vi "Send Text Using SMTP API 2013 NIVerified.vi"(2 "phone number 2":string, 3 "Carrier 2":enum16{"T-Mobile", "AT&T", "Verizon", "Sprint"}(ring), 4 "Body":string, 5 "Carrier 1":enum16{"T-Mobile", "AT&T", "Verizon", "Sprint"}(ring), 6 "Subject":string, 7 "phone number 1":string, 9 "Outgoing Mail Server (SMTP)":string="smtp.gmail.com", 10 "Password":string, 11 "Email":string) -> ()   [LabVIEW 2018]
uses:
  <vilib>/smtpClient/Set Message Text.vi
  <vilib>/smtpClient/LabVIEWSMTPClient.lvlib
panel:
  in  "TLS":bool=TRUE
  # "Overview\nThis example will allows you to use an SMTP server to send a SMS message to a cell phone.\nDescription\nWith the SMTP API you can send an email to your phone as a text message.  There are a lot of different servers you\n can use the default in this example is using GMAIL through the smtp.gmail.com server.  Most SMTP servers should \nwork, but the server and cell phone needs to be compatible to send and receive SMS messages.\nSteps to Implement or Execute Code\nOpen Send Text using SMTP API.vi\nFill in the SMTP server in the Outgoing Mail Server (SMTP), gmail is the default server\nFill out your email & Password\nSelect your Carrier and Type your Phone Number\nType the text you would like to send in the Body Control"
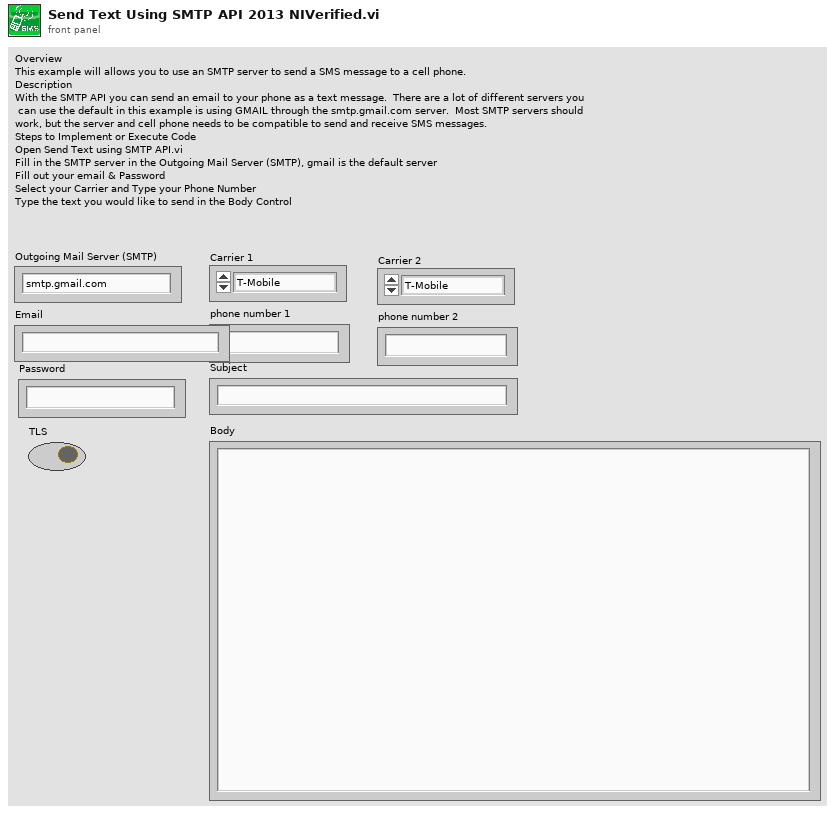
[diagram p1: front panel]
types:
  T1 = typedef "LabVIEWSMTPClient.lvlib/SmtpClientHandle.ctl" = refnum<k1>
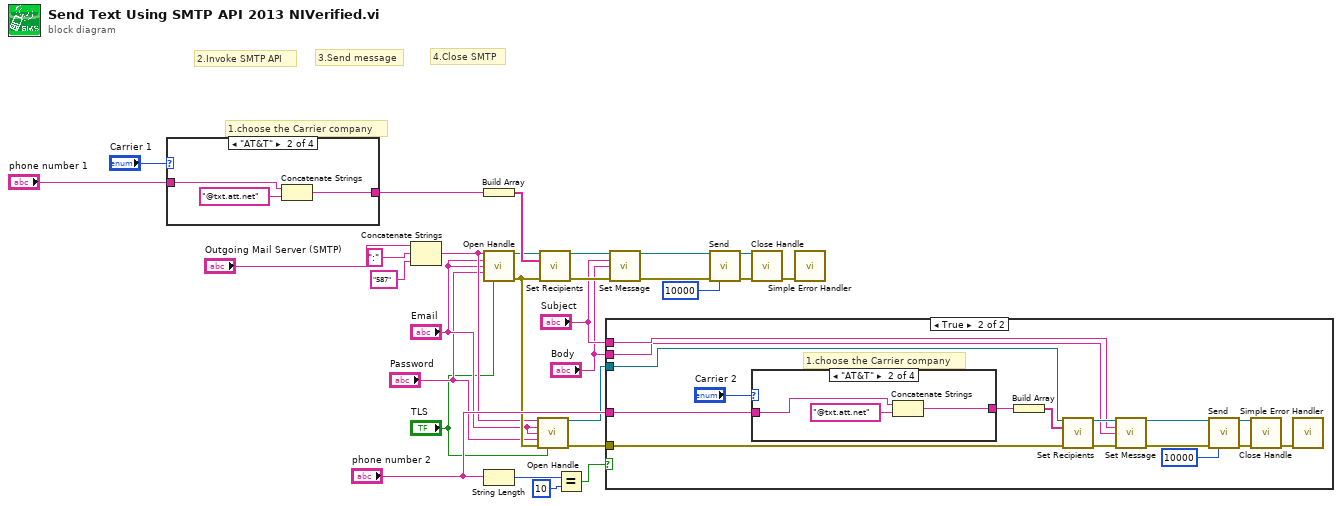
[diagram p0: block diagram]
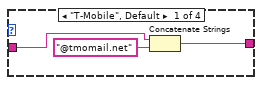
[diagram p3: hidden frame]
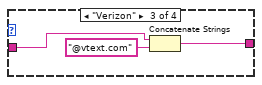
[diagram p4: hidden frame]
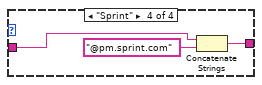
[diagram p5: hidden frame]
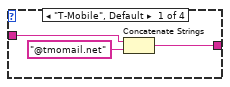
[diagram p6: hidden frame]
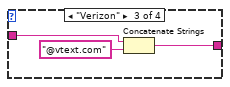
[diagram p7: hidden frame]
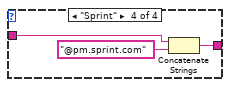
[diagram p8: hidden frame]
diagram:
  # "4.Close SMTP"
  # "3.Send message"
  # "2.Invoke SMTP API"
  # "1.choose the Carrier company"
  n1 = case shown="\"AT&T\"" "Carrier 1" {
    tunnel: "phone number 1" -> [w32 w34 w37 w40]
    tunnel: [w30 w35 w38 w41] -> w21
    frame "T-Mobile", Default {
      n2 = Concatenate Strings(w32, "@tmomail.net" ("string")) -> (w30:string)
    }
    frame "AT&T" {
      n3 = Concatenate Strings(w34, "@txt.att.net" ("string")) -> (w35:string)
    }
    frame "Verizon" {
      n4 = Concatenate Strings(w37, "@vtext.com" ("string")) -> (w38:string)
    }
    frame "Sprint" {
      n5 = Concatenate Strings(w40, "@pm.sprint.com") -> (w41:string)
    }
  }
  n6 = Concatenate Strings("Outgoing Mail Server (SMTP)", ":" ("string"), "587" ("Port")) -> (w5:string)
  n7 = Build Array(w21) -> (w20:string[])
  n8 = call <vilib>:"Open Handle.vi"("server address"=w5, "from"="Email", "username"="Email", "password"="Password", "use TLS (false)"="TLS") -> ("handle out"=w10:T1, "error out"=w7:errorcluster)  [unwired: 9 in]
  n9 = String Length(string="phone number 2") -> (length=w13:i32)
  n10 = call <vilib>:"Open Handle.vi"("server address"=w5, "from"="Email", "username"="Email", "password"="Password", "error in (no error)"=w7, "use TLS (false)"="TLS") -> ("handle out"=w1:T1, "error out"=w6:errorcluster)  [unwired: 8 in]
  n11 = call <vilib>:"Set Recipients.vi"("handle in"=w10, "to"=w20, "error in (no error)"=w7) -> ("handle out"=w27:T1, "error out"=w26:errorcluster)  [unwired: 11 in]
  n12 = Equal?(x=w13, y=10) -> (x = y?=w11:bool)
  n13 = case shown="True" w11 {
    tunnel: "phone number 2" -> [_ w57]
    tunnel: w6 -> [_ w45]
    tunnel: w1 -> [_ w44]
    tunnel: "Subject" -> [_ w43]
    tunnel: "Body" -> [_ w42]
    frame False {
    }
    frame True {
      # "1.choose the Carrier company"
      n14 = case shown="\"AT&T\"" "Carrier 2" {
        tunnel: w57 -> [w60 w62 w65 w68]
        tunnel: [w58 w63 w66 w69] -> w49
        frame "T-Mobile", Default {
          n15 = Concatenate Strings(w60, "@tmomail.net" ("string")) -> (w58:string)
        }
        frame "AT&T" {
          n16 = Concatenate Strings(w62, "@txt.att.net" ("string")) -> (w63:string)
        }
        frame "Verizon" {
          n17 = Concatenate Strings(w65, "@vtext.com" ("string")) -> (w66:string)
        }
        frame "Sprint" {
          n18 = Concatenate Strings(w68, "@pm.sprint.com") -> (w69:string)
        }
      }
      n19 = Build Array(w49) -> (w48:string[])
      n20 = call <vilib>:"Set Recipients.vi"("handle in"=w44, "to"=w48, "error in (no error)"=w45) -> ("handle out"=w55:T1, "error out"=w54:errorcluster)  [unwired: 11 in]
      n21 = call-poly <vilib>:"Set Message.vi"("handle in"=w55, "subject"=w43, "plain text message"=w42, "error in (no error)"=w54) -> ("handle out"=w53:T1, "error out"=w52:errorcluster)  [unwired: 10 in]
      n22 = call <vilib>:"Send.vi"("handle in"=w53, "error in (no error)"=w52, "timeout in ms (10000)"=10000) -> ("handle out"=w51:T1, "error out"=w50:errorcluster)  [unwired: 10 in, 1 out]
      n23 = call <vilib>:"Close Handle.vi"("handle in"=w51, "error in (no error)"=w50) -> ("error out"=w46:errorcluster)  [unwired: 12 in, 1 out]
      n24 = call <vilib>:"Simple Error Handler.vi"("error in (no error)"=w46) -> ()  [unwired: 4 in, 5 out]
    }
  }
  n25 = call-poly <vilib>:"Set Message.vi"("handle in"=w27, "subject"="Subject", "plain text message"="Body", "error in (no error)"=w26) -> ("handle out"=w25:T1, "error out"=w24:errorcluster)  [unwired: 10 in]
  n26 = call <vilib>:"Send.vi"("handle in"=w25, "error in (no error)"=w24, "timeout in ms (10000)"=10000) -> ("handle out"=w23:T1, "error out"=w22:errorcluster)  [unwired: 10 in, 1 out]
  n27 = call <vilib>:"Close Handle.vi"("handle in"=w23, "error in (no error)"=w22) -> ("error out"=w15:errorcluster)  [unwired: 12 in, 1 out]
  n28 = call <vilib>:"Simple Error Handler.vi"("error in (no error)"=w15) -> ()  [unwired: 4 in, 5 out]
